vi "AnalogAQ Canal.vi"(8 "error in":errorcluster, 9 "Numero de Muestras":i32=1000, 10 "Frecuencia":dbl=1000.0 format="%0.2f", 11 "DAQmx Board Name":tag="DAQSim1") -> (0 "error out":errorcluster, 3 "Classic DAQmx Task Name":refnum<k21>)   [LabVIEW 2020]
uses:
  <vilib>/DAQmx/create/channels.llb/DAQmx Create Channel (AI-Voltage-Basic).vi
  <vilib>/DAQmx/configure/timing.llb/DAQmx Timing (Sample Clock).vi
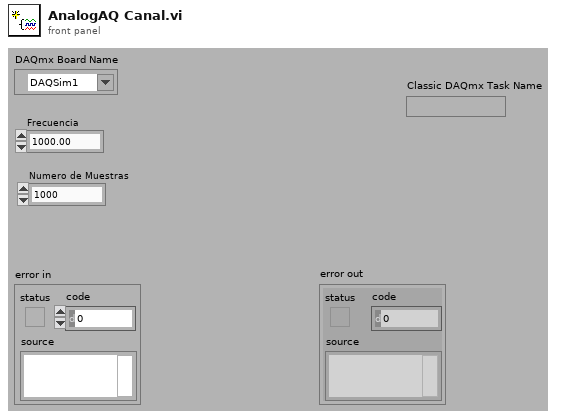
[diagram p1: front panel]
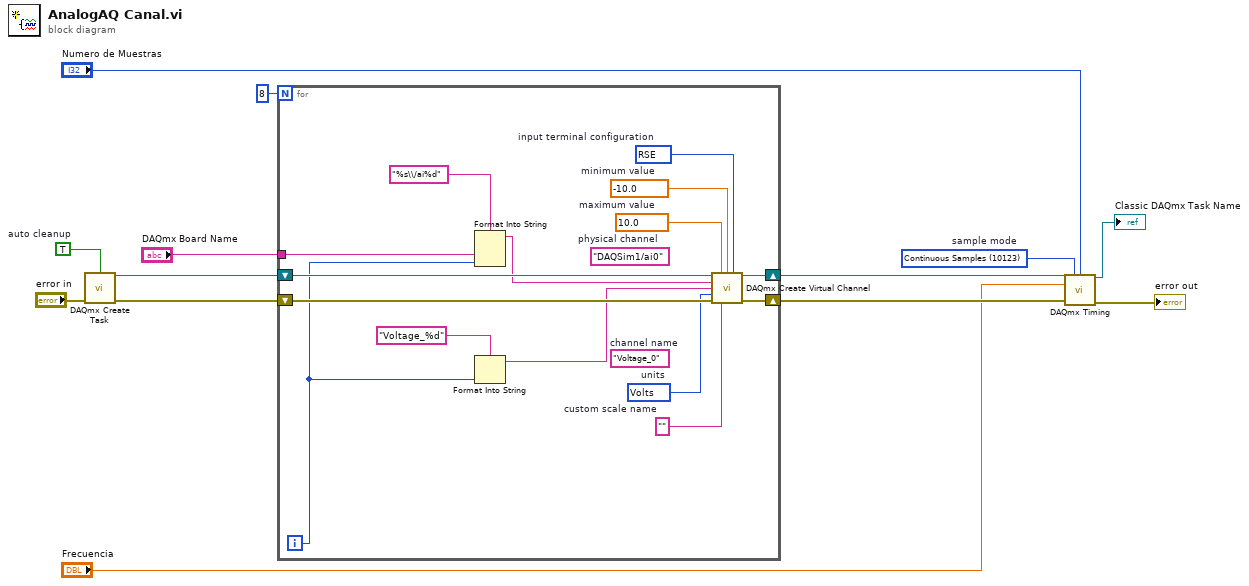
[diagram p0: block diagram]
diagram:
  w6 = 10123 items=["Finite Samples"=10178, "Continuous Samples"=10123, "Hardware Timed Single Point"=12522]  # sample mode
  w11 = TRUE  # auto cleanup
  n1 = call <vilib>:"DAQmx Create Task.vi"("auto cleanup"=w11, "error in"="error in") -> ("task out"=w10:refnum<k21>, "error out"=w12:errorcluster)  [unwired: 12 in]
  n2 = for {
    N: 8 -> [_]
    shift-right: [w23] -> w9
    shift-left: w12 -> [w28]
    shift-right: [w20] -> w8
    shift-left: w10 -> [w27]
    tunnel: "DAQmx Board Name" -> [w15]
    i -> [w14]
    w21 = 10083 items=["default"=-1, "RSE"=10083, "NRSE"=10078, "Differential"=10106, "Pseudodifferential"=12529]  # input terminal configuration
    w22 = 10348 items=["Volts"=10348, "From Custom Scale"=10065]  # units
    (unwired) "Voltage_0"  # channel name
    w24 = ""  # custom scale name
    w25 = -10.0  # minimum value
    w26 = 10.0  # maximum value
    (unwired) "DAQSim1/ai0"  # physical channel
    n3 = Format Into String(format string="%s\\/ai%d", w15, w14) -> (resulting string=w17:string)  [unwired: 2 in, 1 out]
    n4 = Format Into String(format string="Voltage_%d", w14) -> (resulting string=w16:string)  [unwired: 2 in, 1 out]
    n5 = call-poly <vilib>:"DAQmx Create Virtual Channel.vi"("task in"=w27, "maximum value"=w26, "minimum value"=w25, "input terminal configuration"=w21, "physical channels"=w17, "name to assign"=w16, "units"=w22, "error in"=w28, "custom scale name"=w24) -> ("task out"=w20:refnum<k21>, "error out"=w23:errorcluster)  [unwired: 5 in]
  }
  n6 = call-poly <vilib>:"DAQmx Timing.vi"("task/channels in"=w8, "sample mode"=w6, "samples per channel"="Numero de Muestras", "rate"="Frecuencia", "error in"=w9) -> ("task out"=→"Classic DAQmx Task Name":refnum<k21>, "error out"=→"error out":errorcluster)  [unwired: 9 in]
